vi "Prepend Error Message.vi"(8 "error in":errorcluster, 11 "message in":string) -> (0 "error out":errorcluster)   [LabVIEW 2022 SP3]
uses:
  <vilib>/Utility/error.llb/Trim Whitespace One-Sided.vi
  <vilib>/regexp/Match Regular Expression.xnode
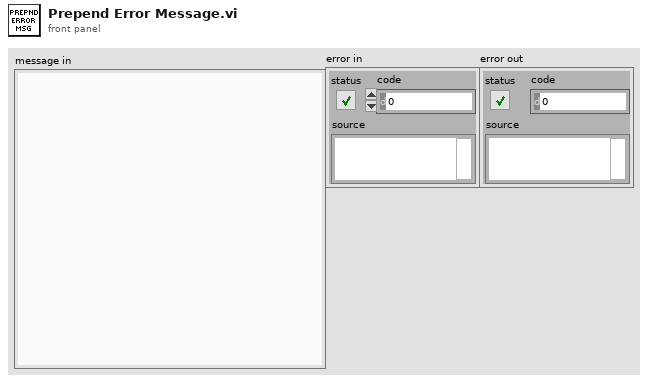
[diagram p1: front panel]
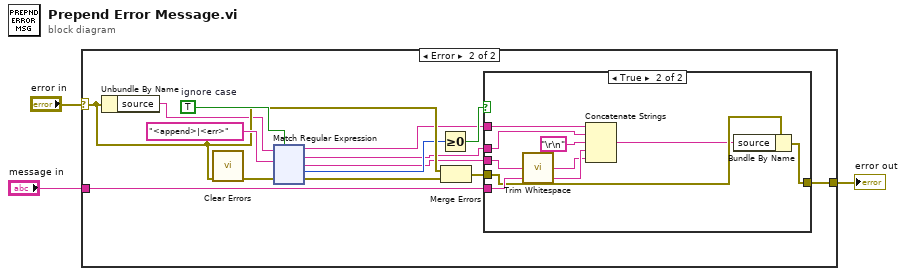
[diagram p0: block diagram]
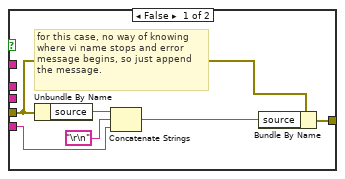
[diagram p3: hidden frame]
diagram:
  n1 = case shown="Error" "error in" {
    selector: "error in" -> [w4 w10]
    tunnel: [w4 w16] -> w3
    tunnel: "message in" -> [_ w17]
    frame No Error {
    }
    frame Error {
      w14 = TRUE  # ignore case
      n2 = Unbundle By Name(w10) -> ("source"=w6:string)
      n3 = call <vilib>:"Clear Errors.vi"("error in (no error)"=w10) -> ("error out"=w13:errorcluster)  [unwired: 5 in, 1 out]
      n4 = xnode "Match Regular Expression"("input string"=w6, "regular expression"="<append>|<err>", "error in"=w13, "ignore case? (F)"=w14) -> ("before match"=w7:string, "whole match"=w5:string, "after match"=w8:string, "offset past match"=w9:i32, "error out"=w12:errorcluster)  [unwired: 2 in]
      n5 = Greater Or Equal To 0?(x=w9) -> (x >= 0?=w18:bool)
      n6 = Merge Errors(w10, w12) -> (w11:errorcluster)
      n7 = case shown="True" w18 {
        tunnel: w5 -> [_ w150]
        tunnel: w17 -> [w136 w149]
        tunnel: w11 -> [w141 w148]
        tunnel: [w140 w147] -> w16
        tunnel: w8 -> [_ w143]
        tunnel: w7 -> [_ w142]
        frame False {
          # "for this case, no way of knowing\nwhere vi name stops and error\nmessage begins, so just append\nthe message."
          n8 = Unbundle By Name(w141) -> ("source"=w139:string)
          n9 = Concatenate Strings(w139, "\r\n", w136) -> (w138:string)
          n10 = Bundle By Name(cluster=w141, "source"=w138) -> (w140:errorcluster)
        }
        frame True {
          n11 = call <vilib>:"Trim Whitespace.vi"("string"=w143) -> ("trimmed string"=w144:string)  [unwired: 1 in]
          n12 = Concatenate Strings(w142, w150, "\r\n", w149, w144) -> (w146:string)
          n13 = Bundle By Name(cluster=w148, "source"=w146) -> (w147:errorcluster)
        }
      }
    }
  }
  "error out" <- w3
